vi "multirateCosimSVPWM.vi"(0 "alpha":sgl, 1 "Parameters":T1={"Deadtime"="Deadtime", "Period"="Period"}, 2 "V_DCLINK":dbl, 5 "beta":sgl, 11 "divider":i32=400) -> (4 "SwitchPositions":T2)   [LabVIEW 2015]
uses:
  SVPWM/SwitchPositions.ctl
  SVPWM/Parameters.ctl
  SVPWM/SVPWM.lvlib
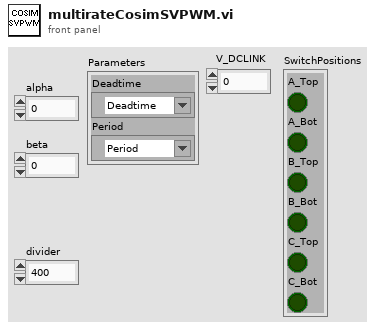
[diagram p1: front panel]
types:
  T1 = typedef "SVPWM.lvlib/Parameters.ctl" = cluster{"Deadtime":refnum<k21>, "Period":refnum<k21>}
  T2 = typedef "SVPWM.lvlib/SwitchPositions.ctl" = cluster{"A_Top":bool, "A_Bot":bool, "B_Top":bool, "B_Bot":bool, "C_Top":bool, "C_Bot":bool}
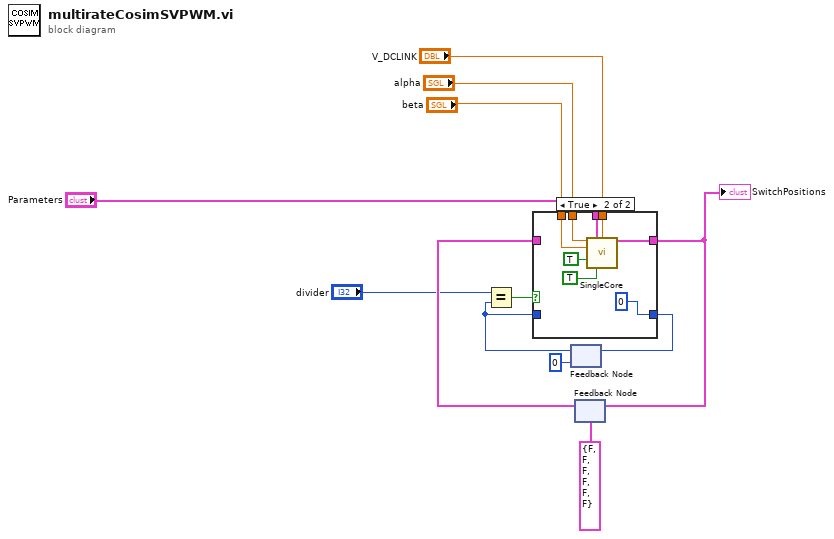
[diagram p0: block diagram]
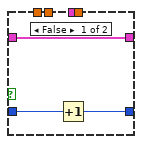
[diagram p2: hidden frame]
diagram:
  n1 = feedback #1 ("Feedback Node 2")(0 ("Constant")) -> (w10:i32)
  n2 = Equal?(x="divider", y=w10) -> (x = y?=w8:bool)
  n3 = feedback #2 ("Feedback Node 3")(T2 {"A_Top"=FALSE, "A_Bot"=FALSE, "B_Top"=FALSE, "B_Bot"=FALSE, "C_Top"=FALSE, "C_Bot"=FALSE} ("SwitchPositions")) -> (w12:T2)
  n4 = case shown="True" w8 {
    tunnel: "Parameters" -> [_ w23]
    tunnel: [w13 w22] -> w11
    tunnel: "V_DCLINK" -> [_ w19]
    tunnel: "alpha" -> [_ w18]
    tunnel: "beta" -> [_ w17]
    tunnel: [w14 0 ("Constant")] -> w7
    tunnel: w10 -> [w15 _]
    tunnel: w12 -> [w13 _]
    frame False {
      n5 = Increment(x=w15) -> (x+1=w14:i32)
    }
    frame True {
      n6 = call "SingleCore.vi"("alpha"=w18, "Parameters"=w23, "ref_max"=w19, "beta"=w17, "input valid"=TRUE, "enable"=TRUE) -> ("SwitchPositions"=w22:T2)  [unwired: 7 in, 2 out]
    }
  }
  "SwitchPositions" <- w11
  n7 = feedback-in #1 ("3")(w7) -> ()
  n8 = feedback-in #2 ("4")(w11) -> ()
